vi "Read Ini File 2012 NIVerified.vi"() -> (1 "Array":dbl[](array[numeric]))   [LabVIEW 2023]
doc: "his example VI shows how to read an ini configuration file and extract all sections, keys, and values from it."
uses:
  <vilib>/Utility/config.llb/Read Key (Double).vi
  <vilib>/Utility/config.llb/NI_LVConfig.lvlib
panel:
  out "keys":string[](array[string])
  out "error out":errorcluster
  in  "error in (no error)":errorcluster
  out "sections":string[](array[string])
  # "Overview:This example VI shows how to read an ini configuration file and extract all sections, keys, and values from it.\nRequirements: \n•\tLabVIEW 2012 (or compatible)\nInstructions:\n1.  (Optional) Save the test file config.ini in a directory on your computer.  You can use any ini file, but this was included for ease of testing.\n2.  Open the attached LabVIEW 2009 vi called read_ini_file.vi.\n3.  In the VI, point to the ini file of choice.\n4.  Run the VI and observe the arrays \"sections\", \"keys\", and \"values\"."
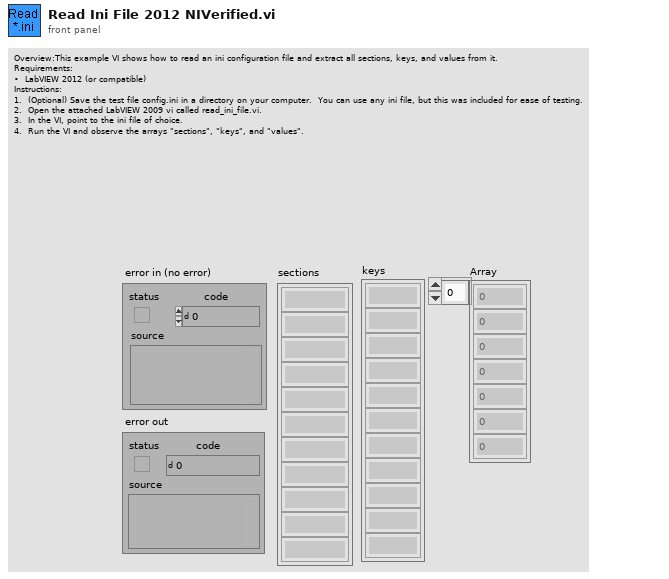
[diagram p1: front panel]
types:
  T1 = typedef "NI_LVConfig.lvlib/Config Data RefNum.ctl" = refnum<k1>
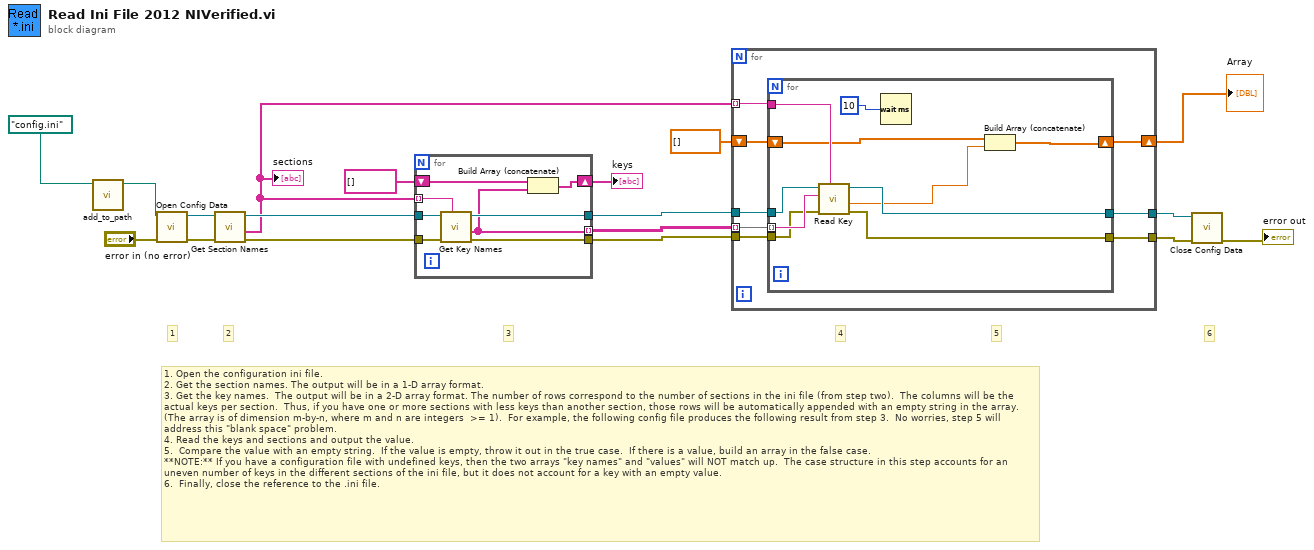
[diagram p0: block diagram]
diagram:
  # "1. Open the configuration ini file.\n2. Get the section names. The output will be in a 1-D array format.\n3. Get the key names.  The output will be in a 2-D array format. The number of rows correspond to the number of sections in the ini file (from step two).  The columns will be the actual keys per section.  Thus, if you have one or more sections with less keys than another section, those rows will be automatically appended with an empty string in the array. (The array is of dimension m-by-n, where m and n are integers  >= 1).  For example, the following config file produces the following result from step 3.  No worries, step 5 will address this \"blank space\" problem.\n4. Read the keys and sections and output the value.\n5.  Compare the value with an empty string.  If the value is empty, throw it out in the true case.  If there is a value, build an array in the false case.\n**NOTE:** If you have a configuration file with undefined keys, then the two arrays \"key names\" and \"values\" will NOT match up.  The case structure in this step accounts for an uneven number of keys in the different sections of the ini file, but it does not account for a key with an empty value.\n6.  Finally, close the reference to the .ini file."
  # "6"
  # "5"
  # "4"
  # "3"
  # "2"
  # "1"
  n1 = call "add_to_path.vi"("Path"=path "config.ini") -> ("appended path"=w2:path)  [unwired: 10 in]
  n2 = call <vilib>:"Open Config Data.vi"("error in (no error)"="error in (no error)", "configuration file path"=w2) -> ("error out"=w18:errorcluster, "refnum"=w17:T1)  [unwired: 7 in, 1 out]
  n3 = call <vilib>:"Get Section Names.vi"("error in (no error)"=w18, "refnum"=w17) -> ("error out"=w15:errorcluster, "section names"=w10:string[], "refnum out"=w16:T1)  [unwired: 7 in]
  "sections" <- w10
  n4 = for {
    tunnel: w16 -> [w26]
    tunnel: w15 -> [w25]
    tunnel: [w24] -> w11
    tunnel: [w23] -> w12
    tunnel: w10 -> [w22] mode=indexing
    shift-right: [w21] -> w8
    shift-left: string[] [] -> [w20]
    tunnel: [w19] -> w7 mode=indexing
    n5 = call <vilib>:"Get Key Names.vi"("section"=w22, "error in (no error)"=w25, "refnum"=w26) -> ("error out"=w24:errorcluster, "key names"=w19:string[], "refnum out"=w23:T1)  [unwired: 5 in, 1 out]
    n6 = Build Array (concatenate)(w20, w19) -> (w21:string[])
  }
  "keys" <- w8
  n7 = for {
    tunnel: w12 -> [w33]
    tunnel: w11 -> [w34]
    tunnel: w10 -> [w32] mode=indexing
    tunnel: w7 -> [w31] mode=indexing
    shift-right: [w30] -> w1
    shift-left: dbl[] [] -> [w29]
    tunnel: [w28] -> w5
    tunnel: [w27] -> w4
    n8 = for {
      tunnel: w33 -> [w42]
      tunnel: w32 -> [w44]
      tunnel: w31 -> [w41] mode=indexing
      tunnel: w34 -> [w40]
      shift-right: [w39] -> w30
      shift-left: w29 -> [w38]
      tunnel: [w37] -> w28
      tunnel: [w36] -> w27
      n9 = call-poly <vilib>:"Read Key.vi"("section"=w44, "error in (no error)"=w40, "key"=w41, "refnum"=w42) -> ("error out"=w36:errorcluster, "value"=w35:dbl, "refnum out"=w37:T1)  [unwired: 4 in, 1 out]
      n10 = Wait (ms)(milliseconds to wait=u32 10) -> ()  [unwired: 1 out]
      n11 = Build Array (concatenate)(w38, w35) -> (w39:dbl[])
    }
  }
  "Array" <- w1
  n12 = call <vilib>:"Close Config Data.vi"("error in (no error)"=w4, "refnum"=w5) -> ("error out"=→"error out":errorcluster)  [unwired: 8 in, 1 out]
